vi "loadETRONdata.vi"() -> ()   [LabVIEW 2012]
uses:
  <vilib>/addons/database/Connection.llb/DB Tools Open Connec (Path).vi
  <vilib>/addons/database/Connection.llb/Conn Execute.vi
  <vilib>/addons/database/Recordset.llb/Rec Fetch Recordset Data (R).vi
  <vilib>/addons/database/Recordset.llb/Rec Destroy - Connection.vi
  <vilib>/addons/database/_DB Variant To Data/Database Variant To Data.xnode
  <vilib>/addons/database/NI_Database_API.lvlib
panel:
  out "Output":string
  in  "working directory":path=path "c:/temp/ETRON"
  out "data":string
  out "error out":errorcluster
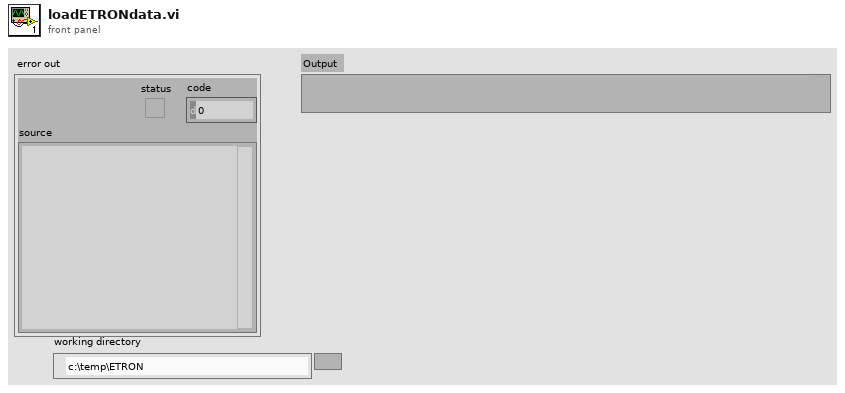
[diagram p1: front panel]
types:
  T1 = typedef "NI_Database_API.lvlib/Conn ObjectReference.ctl" = refnum<k1>
  T2 = typedef "NI_Database_API.lvlib/Rec ObjectReference.ctl" = refnum<k1>
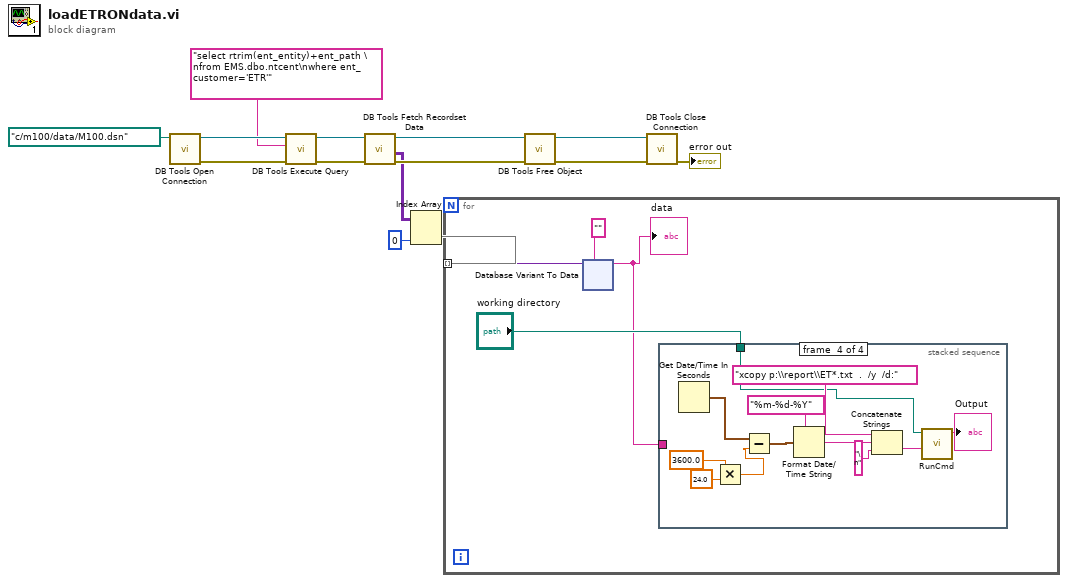
[diagram p0: block diagram]
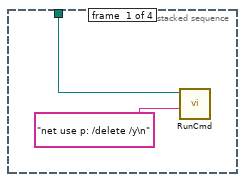
[diagram p2: hidden frame]
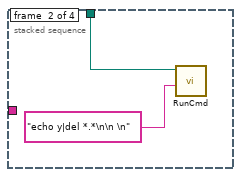
[diagram p3: hidden frame]
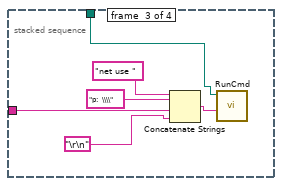
[diagram p4: hidden frame]
diagram:
  n1 = call-poly <vilib>:"DB Tools Open Connection.vi"("connection information"=path "c:/m100/data/M100.dsn") -> ("error out"=w10:errorcluster, "connection reference"=w14:T1)  [unwired: 7 in]
  n2 = call-poly <vilib>:"DB Tools Execute Query.vi"("error in (no error)"=w10, "SQL query"="select rtrim(ent_entity)+ent_path \nfrom EMS.dbo.ntcent\nwhere ent_customer='ETR'", "connection reference"=w14) -> ("error out"=w9:errorcluster, "recordset reference"=w13:T2)  [unwired: 5 in]
  n3 = call-poly <vilib>:"DB Tools Fetch Recordset Data.vi"("error in (no error)"=w9, "recordset reference"=w13) -> ("error out"=w8:errorcluster, "recordset data"=w3:variant[][], "recordset reference out"=w12:T2)  [unwired: 3 in]
  n4 = Index Array(array=w3, index (col)=0 ("disabled index (col)")) -> (element=w1:variant[])  [unwired: 1 in]
  n5 = for {
    tunnel: w1 -> [w18] mode=indexing
    n6 = xnode "Database Variant To Data"("database variant"=w18, "type"="") -> ("data"=w15:string)  [unwired: 1 in, 1 out]
    "data" <- w15
    n7 = stacked-sequence {
      tunnel: "working directory" -> [w19 w21 w24 w29]
      tunnel: w15 -> [_ _ w23 _]
      frame #0 {
        n8 = call "RunCmd.vi"("Cmd String"="net use p: /delete /y\n" ("string"), "working directory"=w19) -> ()  [unwired: 8 in, 2 out]
      }
      frame #1 {
        n9 = call "RunCmd.vi"("Cmd String"="echo y|del *.*\n\n \n" ("standard input"), "working directory"=w21) -> ()  [unwired: 8 in, 2 out]
      }
      frame #2 {
        n10 = Concatenate Strings("net use " ("string"), "p:  \\\\" ("string"), w23, "\r\n") -> (w28:string)
        n11 = call "RunCmd.vi"("Cmd String"=w28, "working directory"=w24) -> ()  [unwired: 8 in, 2 out]
      }
      frame #3 {
        n12 = Get Date/Time In Seconds() -> (seconds since 1Jan1904=w31:timestamp)
        n13 = Multiply(x=3600.0, y=24.0) -> (x*y=w33:dbl)
        n14 = Subtract(x=w31, y=w33) -> (x-y=w34:timestamp)
        n15 = Format Date/Time String(time format string (%c)="%m-%d-%Y", seconds (now)=w34) -> (date/time string=w37:string)  [unwired: 1 in]
        n16 = Concatenate Strings("xcopy p:\\report\\ET*.txt  .  /y  /d:" ("string"), w37, "\n" ("string")) -> (w40:string)
        n17 = call "RunCmd.vi"("Cmd String"=w40, "working directory"=w29) -> ("Output"=→"Output":string)  [unwired: 8 in, 1 out]
      }
    }
  }
  n18 = call-poly <vilib>:"DB Tools Free Object.vi"("error in (no error)"=w8, "recordset reference"=w12) -> ("error out"=w7:errorcluster, "connection reference"=w11:T1)  [unwired: 8 in]
  n19 = call <vilib>:"DB Tools Close Connection.vi"("error in (no error)"=w7, "connection reference"=w11) -> ("error out"=→"error out":errorcluster)  [unwired: 5 in]
